vi "SQL.vi"(8 "error in":errorcluster, 10 "Data":T1) -> (0 "error out":errorcluster, 2 "SQL querry":string)   [LabVIEW 2015]
uses:
  Typedefs/dane.ctl
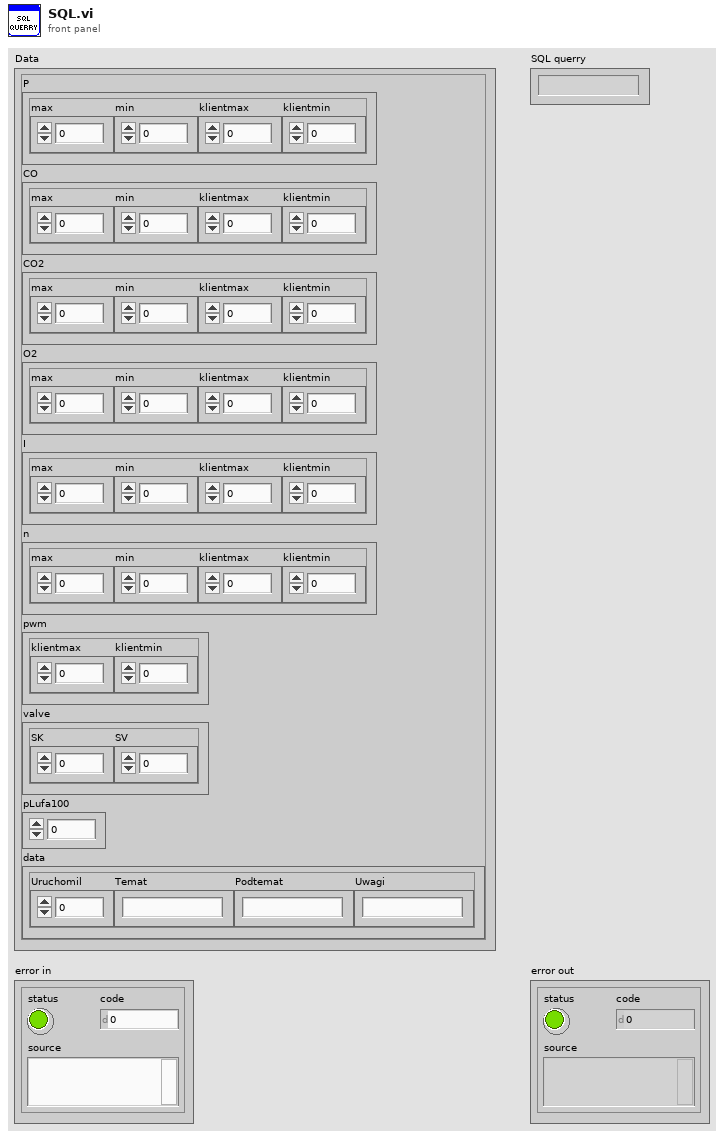
[diagram p1: front panel]
types:
  T1 = typedef "dane.ctl" = cluster{"P":cluster{"max":dbl, "min":dbl, "klientmax":dbl, "klientmin":dbl}, "CO":cluster{"max":dbl, "min":dbl, "klientmax":dbl, "klientmin":dbl}, "CO2":cluster{"max":dbl, "min":dbl, "klientmax":dbl, "klientmin":dbl}, "O2":cluster{"max":dbl, "min":dbl, "klientmax":dbl, "klientmin":dbl}, "I":cluster{"max":dbl, "min":dbl, "klientmax":dbl, "klientmin":dbl}, "n":cluster{"max":dbl, "min":dbl, "klientmax":dbl, "klientmin":dbl}, "pwm":cluster{"klientmax":dbl, "klientmin":dbl}, "valve":cluster{"SK":dbl, "SV":dbl}, "pLufa100":dbl, "data":cluster{"Uruchomil":dbl, "Temat":string, "Podtemat":string, "Uwagi":string}}
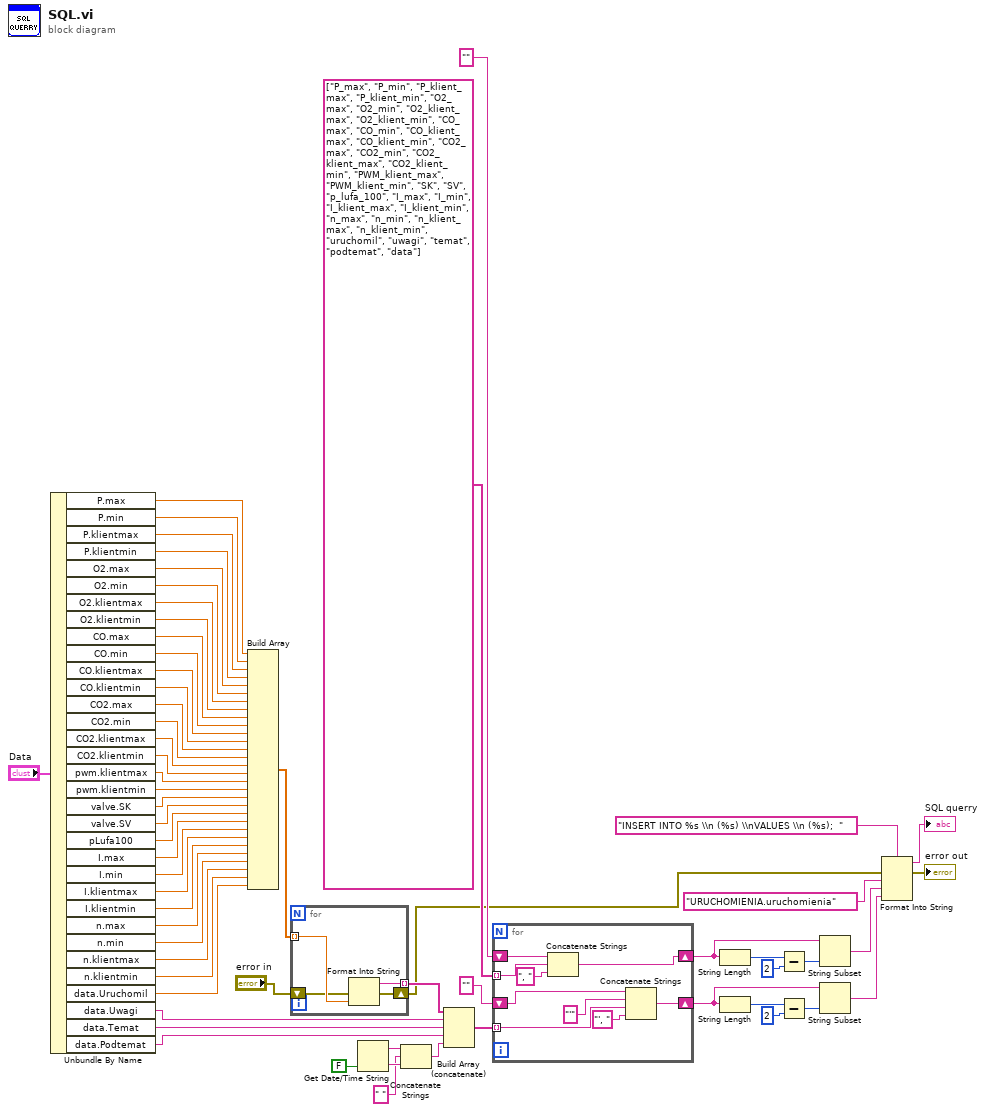
[diagram p0: block diagram]
diagram:
  n1 = Unbundle By Name("Data") -> ("P.max"=w24:dbl, "P.min"=w25:dbl, "P.klientmax"=w26:dbl, "P.klientmin"=w27:dbl, "O2.max"=w28:dbl, "O2.min"=w29:dbl, "O2.klientmax"=w30:dbl, "O2.klientmin"=w31:dbl, "CO.max"=w32:dbl, "CO.min"=w33:dbl, "CO.klientmax"=w34:dbl, "CO.klientmin"=w35:dbl, "CO2.max"=w36:dbl, "CO2.min"=w37:dbl, "CO2.klientmax"=w38:dbl, "CO2.klientmin"=w39:dbl, "pwm.klientmax"=w40:dbl, "pwm.klientmin"=w41:dbl, "valve.SK"=w42:dbl, "valve.SV"=w43:dbl, "pLufa100"=w44:dbl, "I.max"=w45:dbl, "I.min"=w46:dbl, "I.klientmax"=w47:dbl, "I.klientmin"=w48:dbl, "n.max"=w49:dbl, "n.min"=w50:dbl, "n.klientmax"=w51:dbl, "n.klientmin"=w52:dbl, "data.Uruchomil"=w53:dbl, "data.Uwagi"=w56:string, "data.Temat"=w57:string, "data.Podtemat"=w58:string)
  n2 = Build Array(w24, w25, w26, w27, w28, w29, w30, w31, w32, w33, w34, w35, w36, w37, w38, w39, w40, w41, w42, w43, w44, w45, w46, w47, w48, w49, w50, w51, w52, w53) -> (w54:dbl[])
  n3 = for {
    tunnel: w54 -> [w65] mode=indexing
    tunnel: [w64] -> w55 mode=indexing
    shift-right: [w62] -> w1
    shift-left: "error in" -> [w63]
    n4 = Format Into String(error in=w63, w65) -> (resulting string=w64:string, error out=w62:errorcluster)  [unwired: 2 in]
  }
  n5 = Get Date/Time String(want seconds? (F)=FALSE) -> (date string=w6:string, time string=w5:string)  [unwired: 2 in]
  n6 = Concatenate Strings(w6, " " ("string"), w5) -> (w61:string)
  n7 = Build Array (concatenate)(w55, w56, w57, w58, w61) -> (w59:string[])
  n8 = for {
    tunnel: string[] ["P_max", "P_min", "P_klient_max", "P_klient_min", "O2_max", "O2_min", "O2_klient_max", "O2_klient_min", "CO_max", "CO_min", "CO_klient_max", "CO_klient_min", "CO2_max", "CO2_min", "CO2_klient_max", "CO2_klient_min", "PWM_klient_max", "PWM_klient_min", "SK", "SV", "p_lufa_100", "I_max", "I_min", "I_klient_max", "I_klient_min", "n_max", "n_min", "n_klient_max", "n_klient_min", "uruchomil", "uwagi", "temat", "podtemat", "data"] ("columns") -> [w74] mode=indexing
    tunnel: w59 -> [w68] mode=indexing
    shift-right: [w72] -> w22
    shift-left: "" -> [w71]
    shift-right: [w70] -> w60
    shift-left: "" -> [w67]
    n9 = Concatenate Strings(w71, w74, ", " ("string")) -> (w72:string)
    n10 = Concatenate Strings(w67, "'" ("string"), w68, "', " ("string")) -> (w70:string)
  }
  n11 = String Length(string=w22) -> (length=w9:i32)
  n12 = String Length(string=w60) -> (length=w14:i32)
  n13 = Subtract(x=w9, y=2) -> (x-y=w10:i32)
  n14 = Subtract(x=w14, y=2) -> (x-y=w13:i32)
  n15 = String Subset(string=w22, length (rest)=w10) -> (substring=w16:string)  [unwired: 1 in]
  n16 = String Subset(string=w60, length (rest)=w13) -> (substring=w17:string)  [unwired: 1 in]
  n17 = Format Into String(format string="INSERT INTO %s \\n (%s) \\nVALUES \\n (%s);  ", error in=w1, "URUCHOMIENIA.uruchomienia" ("table"), w16, w17) -> (resulting string=→"SQL querry":string, error out=→"error out":errorcluster)  [unwired: 1 in]
